vi "Command (write) - IF.vi"(7 "timeout ms (100)":i32=100, 8 "error in (no error)":errorcluster, 9 "Format":string, 10 "IP":string, 11 "connection ID in":refnum<k16>) -> (0 "error out":errorcluster, 3 "connection ID out":refnum<k16>)   [LabVIEW 2016, in "SMD-7615.lvlib" / "eSCL.lvlib"]
doc: "IF - Immediate Format\nSets the data format, hexadecimal or decimal, for data returned using all “I” commands (except IH, IL, IO and IS).Data can be requested from the drive in two formats: hexadecimal or decimal. By default data is returned in hexadecimal because of its speed and efficiency. Conversion to ascii in the decimal format is slower and causes a slight delay that varies in length. Hexadecimal minimizes the overhead required to convert the internal binary data to ascii form. This speeds up the process of sending out the requested data thus giving the most recent value. Typically, applications written on more powerful host computers can easily convert a hexadecimal value into a decimal value.\nAll “I” commands can be used at any time and at the fastest rate possible limited only by the given baud rate (see BR and PB commands). Immediate commands are executed as they are received, regardless of what is in the drive’s command buffer. Regardless of format (hex or dec) there will be a slight delay in processing the response to an “I” command. “Real time” usage of the data must be carefully analyzed."
uses:
  eSCL.lvlib
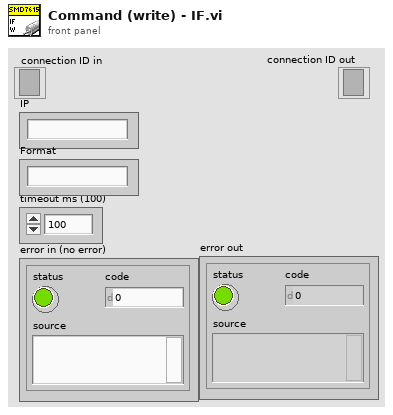
[diagram p1: front panel]
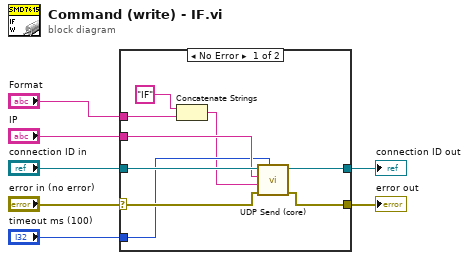
[diagram p0: block diagram]
diagram:
  n1 = case shown="No Error" "error in (no error)" {
    selector: "error in (no error)" -> [w16 w17]
    tunnel: "connection ID in" -> [w15 w18]
    tunnel: [w10 w18] -> w5
    tunnel: [w9 w17] -> w4
    tunnel: "IP" -> [w14 _]
    tunnel: "timeout ms (100)" -> [w13 _]
    tunnel: "Format" -> [w11 _]
    frame No Error {
      n2 = Concatenate Strings("IF" ("Data"), w11) -> (w8:string)
      n3 = call "UDP Send (core).vi"("timeout ms (100)"=w13, "error in (no error)"=w16, "Data"=w8, "IP"=w14, "connection ID in"=w15) -> ("error out"=w9:errorcluster, "connection ID out"=w10:refnum<k16>)  [unwired: 5 in]
    }
    frame Error {
    }
  }
  "connection ID out" <- w5
  "error out" <- w4
